vi "Get Bus Controller.vi"(8 "error in":errorcluster, 11 "1553channel ref in":refnum<k24>) -> (0 "error out":errorcluster, 2 "busController":refnum<k24>, 3 "1553channel ref out":refnum<k24>)   [LabVIEW 2020, in "Ballard_1553_Hardware_ni.lvlib"]
uses:
  Ballard_1553_Hardware_ni.lvlib
  C:/Users/Administrator/Desktop/GIT/Ballard-MIL-STD-1553-Custom-Device/Source/System Explorer/SubVIs/Parse XML Ballard/1.2/BTIXML_SerDes.dll
  Ballard-MIL-STD-1553-Custom-Device/Source/System Explorer/SubVIs/Parse XML Ballard/1.2/BTIXML_SerDes.dll
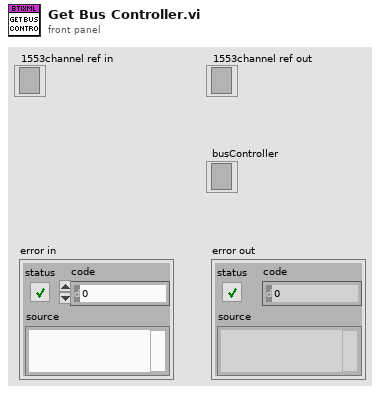
[diagram p1: front panel]
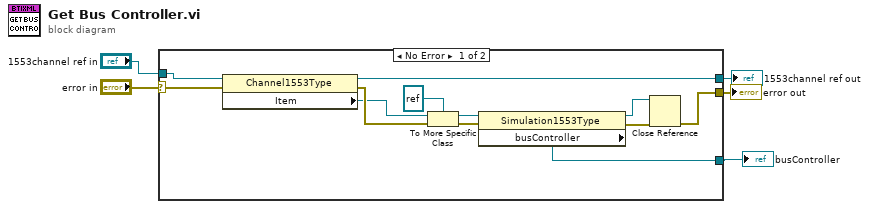
[diagram p0: block diagram]
diagram:
  n1 = case shown="No Error" "error in" {
    selector: "error in" -> [w7 w18]
    tunnel: [w8 w18] -> w5
    tunnel: [w17 w19] -> w4
    tunnel: "1553channel ref in" -> [w16 w19]
    tunnel: [w6 _] -> w1
    frame No Error {
      n2 = property class="Channel1553Type"(reference=w16, error in=w7) -> (reference out=w17:refnum<k24>, error out=w15:errorcluster, "Item"=w14:refnum<k24>)
      n3 = To More Specific Class(target class=refnum<k24> refnum, reference=w14, error in=w15) -> (specific class reference=w12:refnum<k24>, error out=w11:errorcluster)
      n4 = property class="Simulation1553Type"(reference=w12, error in=w11) -> (reference out=w9:refnum<k24>, error out=w10:errorcluster, "busController"=w6:refnum<k24>)
      n5 = Close Reference(reference=w9, error in (no error)=w10) -> (error out=w8:errorcluster)
    }
    frame Error {
    }
  }
  "error out" <- w5
  "1553channel ref out" <- w4
  "busController" <- w1
